vi "Global 1.vi"() -> ()   [LabVIEW 2013]
panel:
  in  "1 48":bool
  in  "1 47":dbl
  in  "1 46":bool
  in  "1 45":dbl
  in  "1 44":bool
  in  "1 43":dbl
  in  "1 42":bool
  in  "1 41":dbl
  in  "1 40":bool
  in  "1 39":dbl
  in  "1 38":bool
  in  "1 37":dbl
  in  "1 36":bool
  in  "1 35":dbl
  in  "1 34":bool
  in  "1 33":dbl
  in  "1 32":bool
  in  "1 31":dbl
  in  "1 30":bool
  in  "1 29":dbl
  in  "1 28":bool
  in  "1 27":dbl
  in  "1 26":bool
  in  "1 25":dbl
  in  "1 24":bool
  in  "1 23":dbl
  in  "1 22":bool
  in  "1 21":dbl
  in  "1 20":bool
  in  "1 19":dbl
  in  "1 18":bool
  in  "1 17":dbl
  in  "1 16":bool
  in  "1 15":dbl
  in  "1 14":bool
  in  "1 13":dbl
  in  "1 12":bool
  in  "1 11":dbl
  in  "1 10":bool
  in  "1 9":dbl
  in  "1 8":bool
  in  "1 7":dbl
  in  "1 6":bool
  in  "1 5":dbl
  in  "1 4":bool
  in  "1 3":dbl
  in  "1 2":bool
  in  "1":dbl
  in  "KD":bool
  in  "KD 2":dbl(slide) scale=0.0..0.3
  in  "KD_vel":bool
  in  "KD_vel 2":dbl(slide) scale=0.0..0.3
  in  "KI_vel":bool
  in  "KP_vel":bool
  in  "KI_vel 2":dbl(slide) scale=0.0..100.0
  in  "KP_vel 2":dbl(slide) scale=0.0..500.0
  in  "KI_ugla":bool
  in  "KP_ugla":bool
  in  "KI_ugla 2":dbl(slide) scale=0.0..100.0
  in  "KP_ugla 2":dbl(slide) scale=0.0..500.0
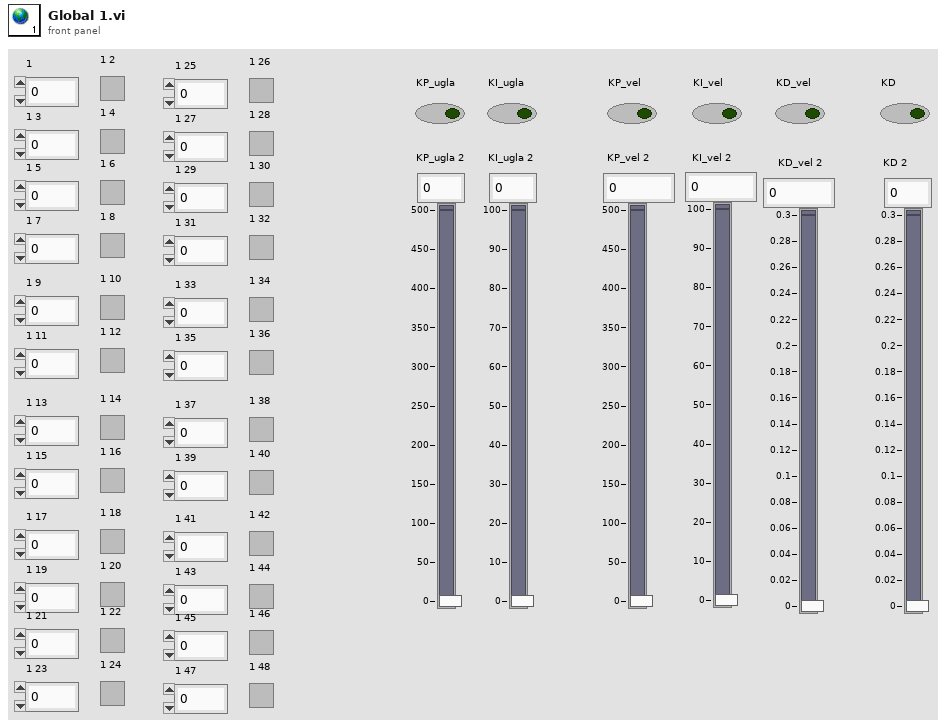
[diagram p1: front panel]
diagram:
